vi "magazine.vi"(9 "Reverse":bool, 10 "Outtake":bool, 11 "Intake":bool) -> ()   [LabVIEW 2020]
uses:
  <vilib>/Rock Robotics/WPI/ThirdParty/Phoenix-LabVIEW/Motor Controller/Controls/CTRE_Phoenix_MotorControl_ControlMode.ctl
  TitanLib/Lib/Piston Hold.vi
  <vilib>/Rock Robotics/WPI/Solenoid/WPI_SolenoidSetEnum.vi
  TitanLib/Lib/TitanLib.lvlib
panel:
  out "Sensor Values":cluster{i16, i16}(graph)
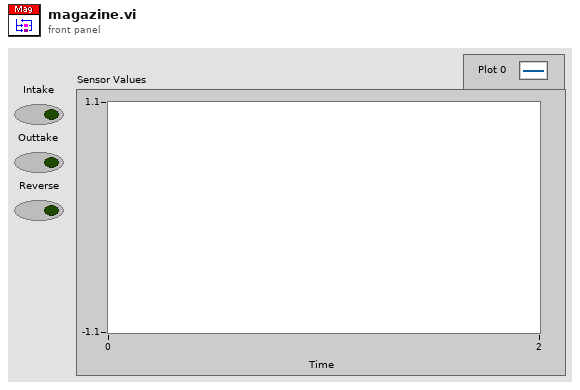
[diagram p1: front panel]
types:
  T1 = typedef "WPI_DigitalInputDevRef.ctl" = cluster{"DevStatus":errorcluster, "DIO Channel":T2}
  T2 = typedef "FPGA_DIOChannel.ctl" = enum8{"DIO 0", "DIO 1", "DIO 2", "DIO 3", "DIO 4", "DIO 5", "DIO 6", "DIO 7", "DIO 8", "DIO 9", "DIO MXP 0", "DIO MXP 1", "DIO MXP 2", "DIO MXP 3", "DIO MXP 4", "DIO MXP 5", "DIO MXP 6", "DIO MXP 7", "DIO MXP 8", "DIO MXP 9", "DIO MXP 10", "DIO MXP 11", "DIO MXP 12", "DIO MXP 13", "DIO MXP 14", "DIO MXP 15", "SPI Port CS1", "SPI Port CS2", "SPI Port CS3", "SPI Port MISO", "SPI Port MOSI", "Invalid"}
  T3 = typedef "WPI_SolenoidValue.ctl" = enum16{"Off", "On", "Forward", "Reverse"}
  T4 = typedef "WPI_SolenoidDevRef.ctl" = cluster{"DevStatus":errorcluster, "Pneumatics Control Module":u8, "Forward Solenoid Channel":T5, "Reverse Solenoid Channel":T5}
  T5 = typedef "WPI_SolenoidChannel.ctl" = enum8{"Solenoid 0", "Solenoid 1", "Solenoid 2", "Solenoid 3", "Solenoid 4", "Solenoid 5", "Solenoid 6", "Solenoid 7", "Solenoid 8", "Solenoid 9", "Solenoid 10", "Solenoid 11", "Solenoid 12", "Solenoid 13", "Solenoid 14", "Solenoid 15", "Invalid"}
  T6 = typedef "CTRE_Phoenix_MotorControl_ControlMode.ctl" = u16
  T7 = typedef "WPI_MotorControlDeviceRef.ctl" = cluster{"DeviceStatus":errorcluster, "Type":T8, "PWM":cluster{"PWM Channel":T9, "DeadBand":T10}, "CAN":cluster{"Device Number":u8, "SetOutput VI Ref":variant, "GetOutput VI Ref":variant, "Enable VI Ref":variant, "Disable VI Ref":variant, "Data":variant}, "Invert":bool, "DIO PWM":cluster{"PWM \"Enable\" Channel":T9, "DIOChannel":T2, "PWM Rate":dbl}}
  T8 = typedef "WPI_MotorControlType.ctl" = enum16{"PWM", "CAN", "DIO PWM"}
  T9 = typedef "FPGA_DIOPWMChannel.ctl" = enum8{"PWM 0", "PWM 1", "PWM 2", "PWM 3", "PWM 4", "PWM 5", "PWM 6", "PWM 7", "PWM 8", "PWM 9", "PWM MXP 0", "PWM MXP 1", "PWM MXP 2", "PWM MXP 3", "PWM MXP 4", "PWM MXP 5", "PWM MXP 6", "PWM MXP 7", "PWM MXP 8", "PWM MXP 9", "Invalid"}
  T10 = typedef "WPI_PWMDeadband.ctl" = cluster{"Name":string, "maxPositivePwm":i32, "minPositivePwm":i32, "centerPwm":i32, "maxNegativePwm":i32, "minNegativePwm":i32, "angularRange":u16}
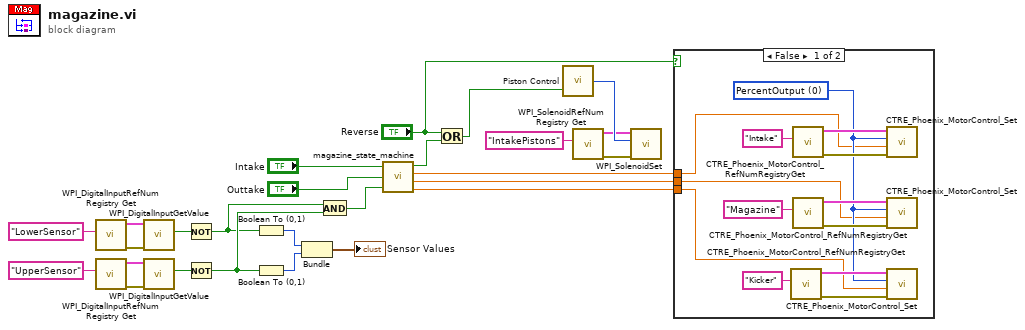
[diagram p0: block diagram]
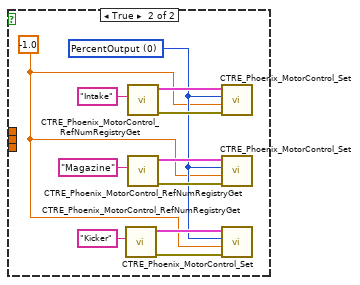
[diagram p2: hidden frame]
diagram:
  n1 = call <vilib>:"WPI_DigitalInputRefNum Registry Get.vi"("refnum name"="LowerSensor") -> ("error out"=w14:errorcluster, "DigitalInputDevRef"=w15:T1)  [unwired: 9 in]
  n2 = call <vilib>:"WPI_DigitalInputRefNum Registry Get.vi"("refnum name"="UpperSensor") -> ("error out"=w11:errorcluster, "DigitalInputDevRef"=w10:T1)  [unwired: 9 in]
  n3 = call <vilib>:"WPI_DigitalInputGetValue.vi"("error in (no error)"=w14, "DigitalInputDevRef"=w15) -> ("Value"=w18:bool)  [unwired: 7 in, 2 out]
  n4 = call <vilib>:"WPI_DigitalInputGetValue.vi"("error in (no error)"=w11, "DigitalInputDevRef"=w10) -> ("Value"=w19:bool)  [unwired: 7 in, 2 out]
  n5 = Not(x=w18) -> (.not. x?=w16:bool)
  n6 = Not(x=w19) -> (.not. x?=w17:bool)
  n7 = Boolean To (0,1)(Boolean=w16) -> (0, 1=w7:i16)
  n8 = Boolean To (0,1)(Boolean=w17) -> (0, 1=w8:i16)
  n9 = Bundle(w7, w8) -> (→"Sensor Values":cluster{i16, i16})  [unwired: 1 in]
  n10 = And(x=w16, y=w17) -> (x .and. y?=w20:bool)
  n11 = call "magazine_state_machine.vi"("Intake Button"="Intake", "Outtake Button"="Outtake", "Both Sensors Active?"=w20) -> ("Intake Pistons"=w24:bool, "Magazine Motor"=w25:dbl, "Intake Motor"=w22:dbl, "Kicker Motor"=w23:dbl)
  n12 = Or(x="Reverse", y=w24) -> (x .or. y?=w6:bool)
  n13 = call-poly "Piston Control.vi"("Input"=w6) -> ("Output"=w5:T3)  [unwired: 1 in]
  n14 = call <vilib>:"WPI_SolenoidRefNum Registry Get.vi"("refnum name"="IntakePistons") -> ("error out"=w2:errorcluster, "SolenoidDevRef"=w3:T4)  [unwired: 9 in]
  n15 = call-poly <vilib>:"WPI_SolenoidSet.vi"("error in (no error)"=w2, "Value"=w5, "SolenoidDevRef"=w3) -> ()  [unwired: 7 in, 2 out]
  n16 = case shown="False" "Reverse" {
    tunnel: w22 -> [w29 _]
    tunnel: w23 -> [w28 _]
    tunnel: w25 -> [w27 _]
    frame False {
      w30 = T6 0 items=["PercentOutput"=0, "Position"=1, "Velocity"=2, "Current"=3, "Follower"=5, "MotionProfile"=6, "MotionMagic"=7, "MotionProfileArc"=10, "Disabled"=15] ("Control Mode")
      n17 = call <vilib>:"CTRE_Phoenix_MotorControl_RefNumRegistryGet.vi"("refnum name"="Kicker") -> ("error out"=w37:errorcluster, "PhoenixMotorControlDevRef"=w36:T7)  [unwired: 9 in]
      n18 = call <vilib>:"CTRE_Phoenix_MotorControl_RefNumRegistryGet.vi"("refnum name"="Intake") -> ("error out"=w39:errorcluster, "PhoenixMotorControlDevRef"=w38:T7)  [unwired: 9 in]
      n19 = call <vilib>:"CTRE_Phoenix_MotorControl_RefNumRegistryGet.vi"("refnum name"="Magazine") -> ("error out"=w34:errorcluster, "PhoenixMotorControlDevRef"=w35:T7)  [unwired: 9 in]
      n20 = call <vilib>:"CTRE_Phoenix_MotorControl_Set.vi"("error in (no error)"=w39, "Output"=w27, "Control Mode"=w30, "PhoenixMotorControlDevRef"=w38) -> ()  [unwired: 6 in, 2 out]
      n21 = call <vilib>:"CTRE_Phoenix_MotorControl_Set.vi"("error in (no error)"=w34, "Output"=w29, "Control Mode"=w30, "PhoenixMotorControlDevRef"=w35) -> ()  [unwired: 6 in, 2 out]
      n22 = call <vilib>:"CTRE_Phoenix_MotorControl_Set.vi"("error in (no error)"=w37, "Output"=w28, "Control Mode"=w30, "PhoenixMotorControlDevRef"=w36) -> ()  [unwired: 6 in, 2 out]
    }
    frame True {
      w40 = -1.0 ("Output")
      w41 = T6 0 items=["PercentOutput"=0, "Position"=1, "Velocity"=2, "Current"=3, "Follower"=5, "MotionProfile"=6, "MotionMagic"=7, "MotionProfileArc"=10, "Disabled"=15] ("Control Mode")
      n23 = call <vilib>:"CTRE_Phoenix_MotorControl_RefNumRegistryGet.vi"("refnum name"="Kicker") -> ("error out"=w48:errorcluster, "PhoenixMotorControlDevRef"=w47:T7)  [unwired: 9 in]
      n24 = call <vilib>:"CTRE_Phoenix_MotorControl_RefNumRegistryGet.vi"("refnum name"="Intake") -> ("error out"=w50:errorcluster, "PhoenixMotorControlDevRef"=w49:T7)  [unwired: 9 in]
      n25 = call <vilib>:"CTRE_Phoenix_MotorControl_RefNumRegistryGet.vi"("refnum name"="Magazine") -> ("error out"=w45:errorcluster, "PhoenixMotorControlDevRef"=w46:T7)  [unwired: 9 in]
      n26 = call <vilib>:"CTRE_Phoenix_MotorControl_Set.vi"("error in (no error)"=w50, "Output"=w40, "Control Mode"=w41, "PhoenixMotorControlDevRef"=w49) -> ()  [unwired: 6 in, 2 out]
      n27 = call <vilib>:"CTRE_Phoenix_MotorControl_Set.vi"("error in (no error)"=w45, "Output"=w40, "Control Mode"=w41, "PhoenixMotorControlDevRef"=w46) -> ()  [unwired: 6 in, 2 out]
      n28 = call <vilib>:"CTRE_Phoenix_MotorControl_Set.vi"("error in (no error)"=w48, "Output"=w40, "Control Mode"=w41, "PhoenixMotorControlDevRef"=w47) -> ()  [unwired: 6 in, 2 out]
    }
  }
